vi "Get LV Path.vi"() -> (0 "String":string)   [LabVIEW 2018, in "Path and String Processing.lvlib"]
uses:
  Path and String Processing.lvlib
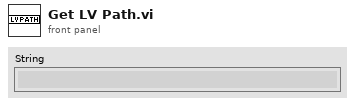
[diagram p1: front panel]
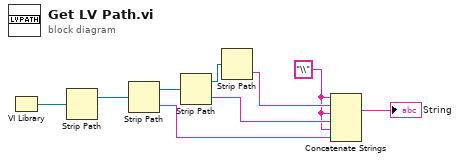
[diagram p0: block diagram]
diagram:
  w2 = "\\" ("string")
  n1 = VI Library() -> (path=w6:path)
  n2 = Strip Path(path=w6) -> (stripped path=w7:path)  [unwired: 1 out]
  n3 = Strip Path(path=w7) -> (stripped path=w8:path, name=w1:string)
  n4 = Strip Path(path=w8) -> (stripped path=w5:path, name=w3:string)
  n5 = Strip Path(path=w5) -> (name=w4:string)  [unwired: 1 out]
  n6 = Concatenate Strings(w2, w4, w2, w3, w2, w1) -> (→"String":string)
